vi "7.2.vi"() -> ()   [LabVIEW 2017]
panel:
  out "波形图":cluster{dbl[]}[](graph)
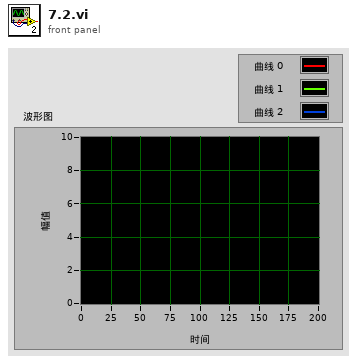
[diagram p1: front panel]
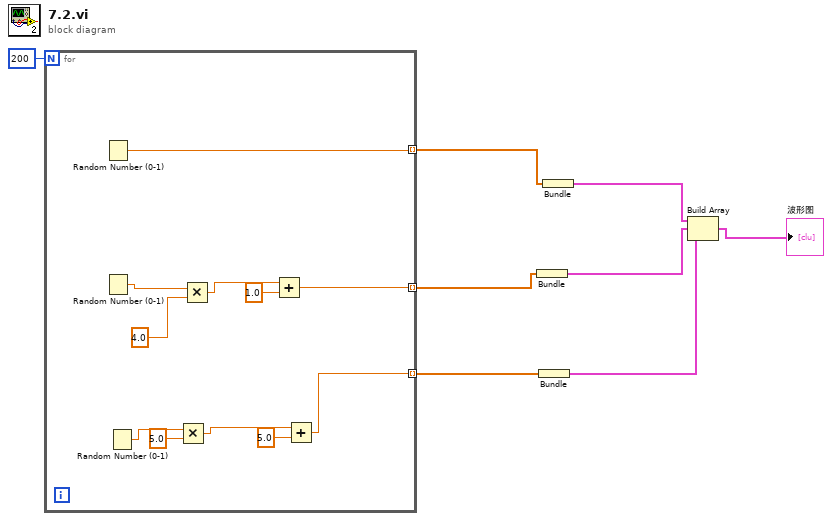
[diagram p0: block diagram]
diagram:
  n1 = for {
    N: 200 -> [_]
    tunnel: [w19] -> w8 mode=indexing
    tunnel: [w18] -> w7 mode=indexing
    tunnel: [w17] -> w6 mode=indexing
    n2 = Random Number (0-1)() -> (number: 0 to 1=w19:dbl)
    n3 = Random Number (0-1)() -> (number: 0 to 1=w16:dbl)
    n4 = Random Number (0-1)() -> (number: 0 to 1=w12:dbl)
    n5 = Multiply(x=w12, y=5.0) -> (x*y=w10:dbl)
    n6 = Multiply(x=w16, y=4.0) -> (x*y=w14:dbl)
    n7 = Add(x=w14, y=1.0) -> (x+y=w18:dbl)
    n8 = Add(x=w10, y=5.0) -> (x+y=w17:dbl)
  }
  n9 = Bundle(w7) -> (w4:cluster{dbl[]})  [unwired: 1 in]
  n10 = Bundle(w6) -> (w3:cluster{dbl[]})  [unwired: 1 in]
  n11 = Bundle(w8) -> (w5:cluster{dbl[]})  [unwired: 1 in]
  n12 = Build Array(w5, w4, w3) -> (→"波形图":cluster{dbl[]}[])
